vi "Agilent SNA IDN INI File.vi"(8 "error in (no error)":errorcluster, 10 "Operation":enum16{"Read", "Write", "Clear"}(ring), 11 "Instrument Info":T1) -> (0 "error out":errorcluster {"code" format="%.0x"}, 2 "Found?":bool, 3 "Instrument Info":T1)   [LabVIEW 2011]
uses:
  TypeDefs/Agilent SNA Instrument Info.ctl
  <vilib>/Utility/config.llb/Read Key (String).vi
  <vilib>/Utility/config.llb/Write Key (String).vi
  <vilib>/Utility/config.llb/NI_LVConfig.lvlib
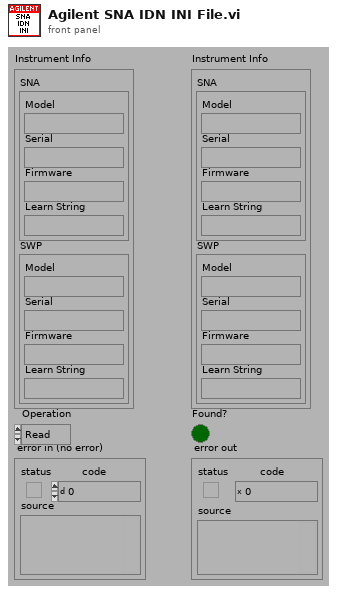
[diagram p1: front panel]
types:
  T1 = typedef "Agilent SNA Instrument Info.ctl" = cluster{"SNA":cluster{"Model":string, "Serial":string, "Firmware":string, "Learn String":string}, "SWP":cluster{"Model":string, "Serial":string, "Firmware":string, "Learn String":string}}
  T2 = typedef "NI_LVConfig.lvlib/Config Data RefNum.ctl" = refnum<k1>
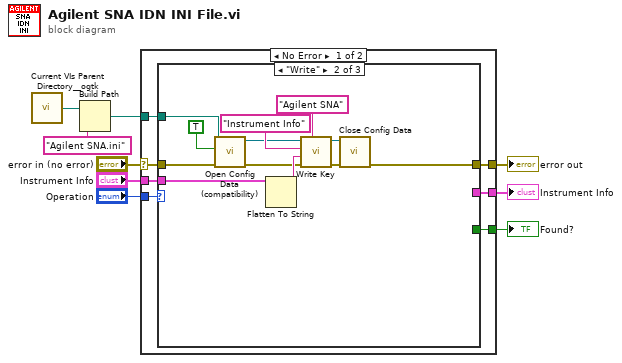
[diagram p0: block diagram]
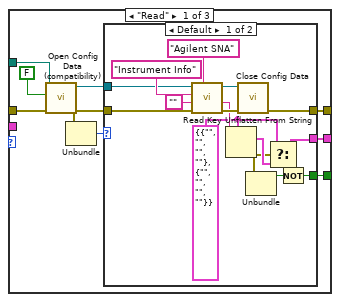
[diagram p2: hidden frame]
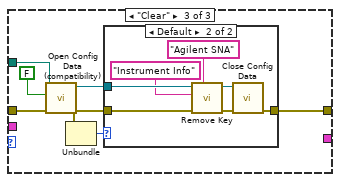
[diagram p4: hidden frame]
diagram:
  n1 = call "Current VIs Parent Directory__ogtk.vi"() -> ("Parent Directory (+ Relative)"=w1:path)  [unwired: 5 in]
  n2 = Build Path(base path=w1, name or relative path="Agilent SNA.ini") -> (appended path=w8:path)
  n3 = case shown="No Error" "error in (no error)" {
    selector: "error in (no error)" -> [w11 w67]
    tunnel: w8 -> [w16 _]
    tunnel: [w15 w67] -> w7
    tunnel: [w14 _] -> w3
    tunnel: "Operation" -> [w13 _]
    tunnel: "Instrument Info" -> [w12 _]
    tunnel: [w10 _] -> w2
    frame No Error {
      n4 = case shown="\"Write\"" w13 {
        tunnel: w16 -> [w22 w43 w55]
        tunnel: w11 -> [w21 w44 w54]
        tunnel: [w25 w42 w53] -> w15
        tunnel: [w24 _ _] -> w14
        tunnel: w12 -> [_ w41 _]
        tunnel: [w17 _ _] -> w10
        frame "Read" {
          n5 = call <vilib>:"Open Config Data (compatibility).vi"("error in (no error)"=w21, "create file if necessary (T)"=FALSE ("create file if necessary? (T)"), "configuration file path"=w22) -> ("error out"=w20:errorcluster, "refnum"=w23:T2)  [unwired: 6 in, 1 out]
          n6 = Unbundle(w20) -> ("code"=w19:i32)  [unwired: 2 out]
          n7 = case shown="Default" w19 {
            tunnel: w20 -> [w33 _]
            tunnel: [w40 _] -> w25
            tunnel: w23 -> [w32 _]
            tunnel: [w30 _] -> w24
            tunnel: [w26 _] -> w17
            frame Default {
              w29 = T1 {"SNA"={"Model"="", "Serial"="", "Firmware"="", "Learn String"=""}, "SWP"={"Model"="", "Serial"="", "Firmware"="", "Learn String"=""}} ("Agilent SNA")
              n8 = call-poly <vilib>:"Read Key.vi"("section"="Agilent SNA" ("name or relative path"), "error in (no error)"=w33, "default value"="", "key"="Instrument Info" ("format string"), "refnum"=w32) -> ("error out"=w37:errorcluster, "value"=w35:string, "refnum out"=w38:T2)  [unwired: 1 in, 3 out]
              n9 = Unflatten From String(type=w29, binary string=w35) -> (value=w31:T1, error out=w28:errorcluster)  [unwired: 1 in, 3 out]
              n10 = call <vilib>:"Close Config Data.vi"("error in (no error)"=w37, "refnum"=w38) -> ("error out"=w40:errorcluster)  [unwired: 1 in, 8 out]
              n11 = Unbundle(w28) -> ("status"=w27:bool)  [unwired: 2 out]
              n12 = Select(t=w29, s=w28, f=w31) -> (s? t:f=w30:T1)
              n13 = Not(x=w27) -> (.not. x?=w26:bool)
            }
            frame 7 {
            }
          }
        }
        frame "Write" {
          n14 = call <vilib>:"Open Config Data (compatibility).vi"("error in (no error)"=w44, "create file if necessary (T)"=TRUE ("create file if necessary? (T)"), "configuration file path"=w43) -> ("error out"=w46:errorcluster, "refnum"=w47:T2)  [unwired: 6 in, 1 out]
          n15 = Flatten To String(anything=w41) -> (data string=w51:string)  [unwired: 1 in, 4 out]
          n16 = call-poly <vilib>:"Write Key.vi"("section"="Agilent SNA", "error in (no error)"=w46, "value"=w51, "key"="Instrument Info" ("format string"), "refnum"=w47) -> ("error out"=w49:errorcluster, "refnum out"=w50:T2)  [unwired: 1 in, 4 out]
          n17 = call <vilib>:"Close Config Data.vi"("error in (no error)"=w49, "refnum"=w50) -> ("error out"=w42:errorcluster)  [unwired: 1 in, 8 out]
        }
        frame "Clear" {
          n18 = call <vilib>:"Open Config Data (compatibility).vi"("error in (no error)"=w54, "create file if necessary (T)"=FALSE ("create file if necessary? (T)"), "configuration file path"=w55) -> ("error out"=w57:errorcluster, "refnum"=w59:T2)  [unwired: 6 in, 1 out]
          n19 = Unbundle(w57) -> ("code"=w56:i32)  [unwired: 2 out]
          n20 = case shown="Default" w56 {
            tunnel: w57 -> [_ w66]
            tunnel: w59 -> [_ w65]
            tunnel: [_ w64] -> w53
            frame 7 {
            }
            frame Default {
              n21 = call <vilib>:"Remove Key.vi"("section"="Agilent SNA" ("name or relative path"), "error in (no error)"=w66, "key"="Instrument Info" ("name or relative path"), "refnum"=w65) -> ("error out"=w61:errorcluster, "refnum out"=w60:T2)  [unwired: 6 out]
              n22 = call <vilib>:"Close Config Data.vi"("error in (no error)"=w61, "refnum"=w60) -> ("error out"=w64:errorcluster)  [unwired: 1 in, 8 out]
            }
          }
        }
      }
    }
    frame Error {
    }
  }
  "error out" <- w7
  "Instrument Info" <- w3
  "Found?" <- w2
